vi "Read INI File.vi"(8 "error in (no error)":errorcluster, 11 "name or relative path":path) -> (0 "error out":errorcluster, 3 "Ini File":T1(array[cluster]))   [LabVIEW 2021]
uses:
  <vilib>/Utility/config.llb/Read Key (U32).vi
  <vilib>/Utility/config.llb/NI_LVConfig.lvlib
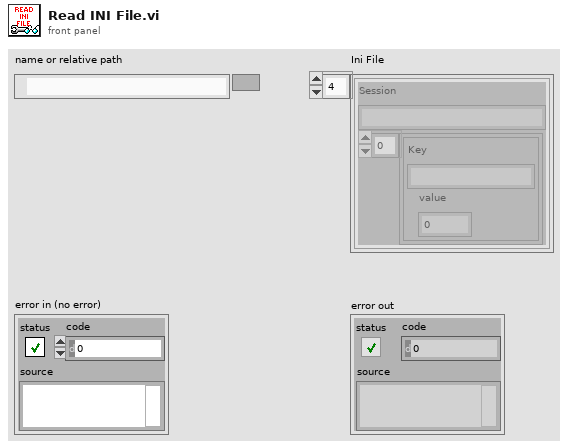
[diagram p1: front panel]
types:
  T1 = cluster{"Session":string, cluster{"Key":string, "value":u32}[]}[]
  T2 = typedef "NI_LVConfig.lvlib/Config Data RefNum.ctl" = refnum<k1>
  T3 = cluster{"String":string, cluster{"String":string, "value":u32}[]}
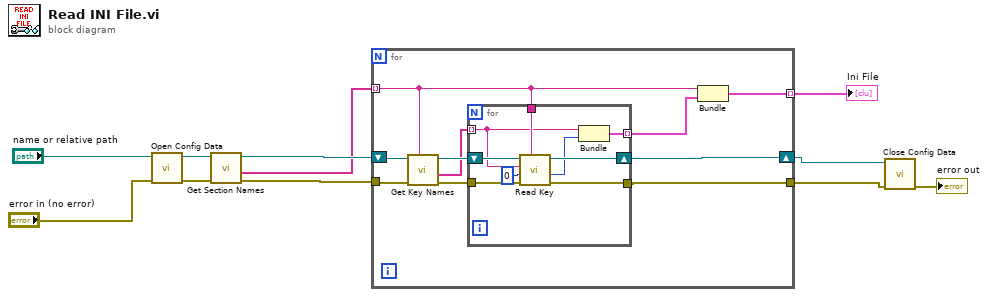
[diagram p0: block diagram]
diagram:
  n1 = call <vilib>:"Open Config Data.vi"("error in (no error)"="error in (no error)", "configuration file path"="name or relative path") -> ("error out"=w8:errorcluster, "refnum"=w9:T2)  [unwired: 7 in, 1 out]
  n2 = call <vilib>:"Get Section Names.vi"("error in (no error)"=w8, "refnum"=w9) -> ("error out"=w6:errorcluster, "section names"=w5:string[], "refnum out"=w7:T2)  [unwired: 7 in]
  n3 = for {
    shift-right: [w16] -> w4
    shift-left: w7 -> [w21]
    tunnel: w6 -> [w20]
    tunnel: w5 -> [w18] mode=indexing
    tunnel: [w19] -> w1 mode=indexing
    tunnel: [w12] -> w3
    n4 = call <vilib>:"Get Key Names.vi"("section"=w18, "error in (no error)"=w20, "refnum"=w21) -> ("error out"=w15:errorcluster, "key names"=w14:string[], "refnum out"=w17:T2)  [unwired: 5 in, 1 out]
    n5 = for {
      tunnel: w18 -> [w30]
      tunnel: w15 -> [w27]
      shift-right: [w28] -> w16
      shift-left: w17 -> [w29]
      tunnel: w14 -> [w24] mode=indexing
      tunnel: [w23] -> w13 mode=indexing
      tunnel: [w22] -> w12
      n6 = call-poly <vilib>:"Read Key.vi"("section"=w30, "error in (no error)"=w27, "default value"=u32 0, "key"=w24, "refnum"=w29) -> ("error out"=w22:errorcluster, "value"=w25:u32, "refnum out"=w28:T2)  [unwired: 3 in, 1 out]
      n7 = Bundle("String"=w24, "value"=w25) -> (w23:cluster{"String":string, "value":u32})  [unwired: 1 in]
    }
    n8 = Bundle("String"=w18, w13) -> (w19:T3)  [unwired: 1 in]
  }
  "Ini File" <- w1
  n9 = call <vilib>:"Close Config Data.vi"("error in (no error)"=w3, "refnum"=w4) -> ("error out"=→"error out":errorcluster)  [unwired: 8 in, 1 out]
